vi "updateLastValues.vi"(6 "last_iterm":dbl, 7 "last_dterm":dbl, 8 "error in (no error)":errorcluster, 9 "last_error":dbl, 10 "last_pterm":dbl, 11 "PIDController in":refnum<class "PIDController.lvclass">) -> (0 "error out":errorcluster, 3 "PIDController out":refnum<class "PIDController.lvclass">)   [LabVIEW 2025, in "PIDController.lvclass"]
uses:
  PIDController.lvclass
  PIDController.lvclass/PIDController.ctl
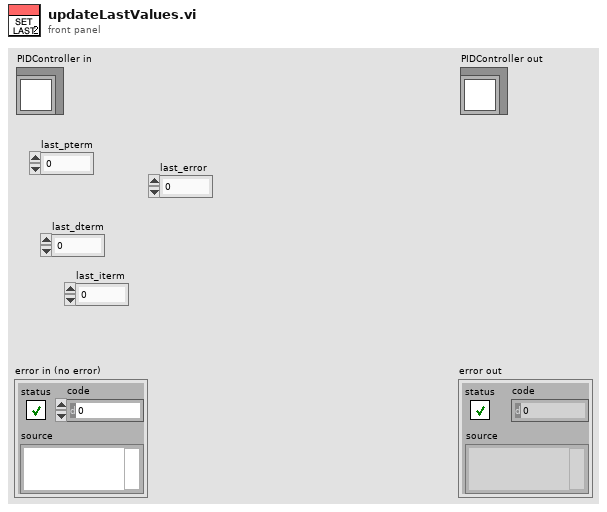
[diagram p1: front panel]
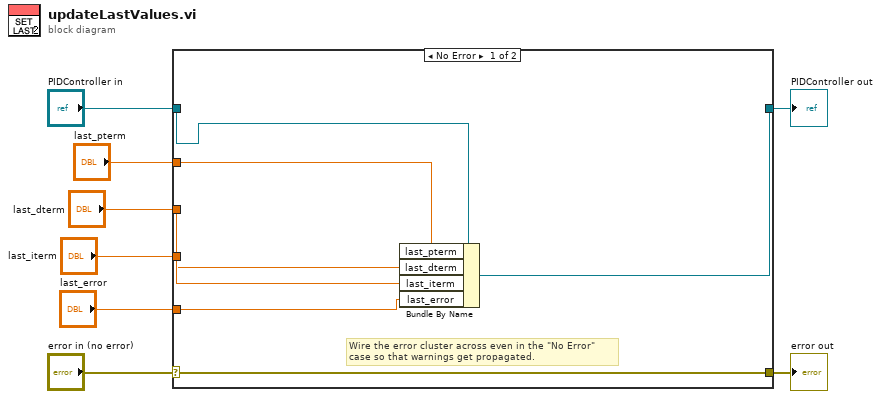
[diagram p0: block diagram]
diagram:
  n1 = case shown="No Error" "error in (no error)" {
    selector: "error in (no error)" -> [w15 w17]
    tunnel: [w15 w17] -> w7
    tunnel: [w13 w16] -> w5
    tunnel: "PIDController in" -> [w14 w16]
    tunnel: "last_pterm" -> [w12 _]
    tunnel: "last_dterm" -> [w9 _]
    tunnel: "last_iterm" -> [w10 _]
    tunnel: "last_error" -> [w11 _]
    frame No Error {
      # "Wire the error cluster across even in the \"No Error\"\ncase so that warnings get propagated."
      n2 = Bundle By Name(cluster=w14, "last_pterm"=w12, "last_dterm"=w9, "last_iterm"=w10, "last_error"=w11) -> (w13:refnum<class "PIDController.lvclass">)
    }
    frame Error {
    }
  }
  "error out" <- w7
  "PIDController out" <- w5
